vi "setExptParam.vi"(8 "error in (no error)":errorcluster, 9 "value":variant, 10 "key":string, 11 "Inst.Transport in":refnum<class "Inst.Transport.lvclass">) -> (0 "error out":errorcluster, 3 "Inst.Transport out":refnum<class "Inst.Transport.lvclass">)   [LabVIEW 2019, in "Inst.Transport.lvclass"]
uses:
  Inst.Transport.lvclass
  Typedefs/Inst.Transport.PublicCommands--Enum.ctl
  <userlib>/LevyLab/LV-Data/LV-Data/Typedefs/Dictionary--cluster.ctl
  <userlib>/LevyLab/LV-Data/LV-Data/LV-Data.lvclass
  Typedefs/setExptParam--Request--Cluster.ctl
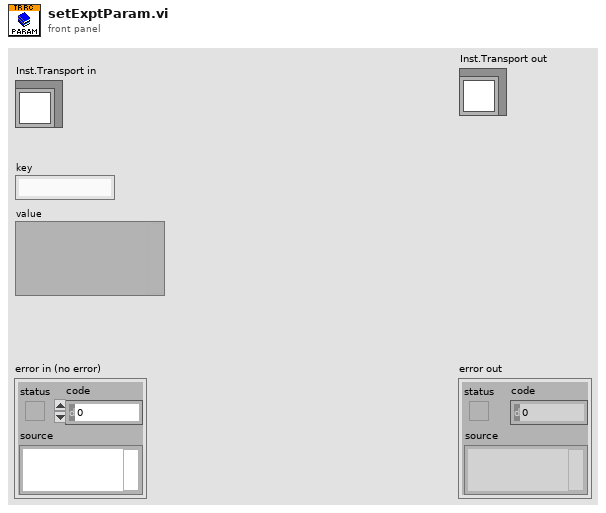
[diagram p1: front panel]
types:
  T1 = typedef "Inst.Transport.lvclass/setExptParam--Request--Cluster.ctl" = cluster{"param":T2}
  T2 = typedef "LV-Data.lvclass/Dictionary--cluster.ctl" = cluster{"key":string, "value":variant}
  T3 = typedef "Inst.Transport.lvclass/Inst.Transport.PublicCommands--Enum.ctl" = enum16{"startTransport", "stopTransport", "setExptFolder", "setExptComments", "appendExptParam", "clearExptParam", "setExptParam", "setSweepConfig"}
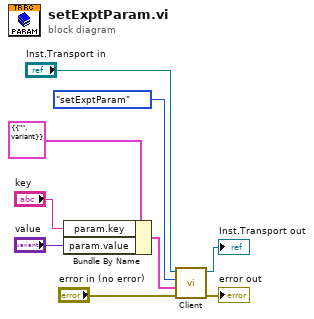
[diagram p0: block diagram]
diagram:
  n1 = Bundle By Name(cluster=T1 {"param"={"key"="", "value"=variant}} ("setExptParam"), "param.key"="key", "param.value"="value") -> (w4:T1)
  n2 = call-dynamic "Client.vi"("error in (no error)"="error in (no error)", "Data in"=w4, "Command in"=Inst.Transport.PublicCommands--Enum."setExptParam" ("Commands"), "Instrument in"="Inst.Transport in") -> ("error out"=→"error out":errorcluster, "Instrument out"=→"Inst.Transport out":refnum<class "Inst.Transport.lvclass">)  [unwired: 4 in, 2 out]
